vi "Read Self ID.vi"(11 "Properties in":refnum<class "Properties.lvclass">) -> (2 "self-id":string, 3 "Properties out":refnum<class "Properties.lvclass">)   [LabVIEW 2020, in "Caraya.lvlib" / "Properties.lvclass"]
uses:
  Properties.lvclass
  Properties.lvclass/Properties.ctl
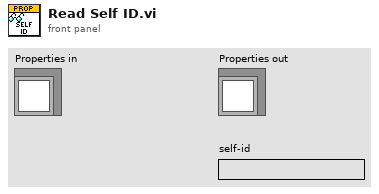
[diagram p1: front panel]
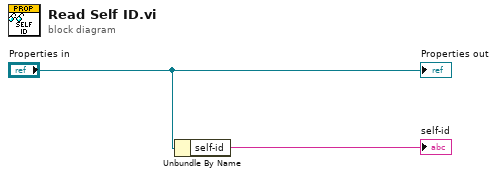
[diagram p0: block diagram]
diagram:
  n1 = Unbundle By Name("Properties in") -> ("self-id"=→"self-id":string)
  "Properties out" <- "Properties in"
